vi "ReadBAESdataFromFileVer3.vi"(2 "Factor Size Parameter":dbl=1.0, 3 "Factor Extinction":dbl=1.0 min=0.0 max=150.0 step=1.0, 4 "Factor Ext Uncertainty":dbl=1.0 min=0.0 max=150.0 step=1.0, 5 "file path":path) -> (0 "Extinction data in graph format":T2(array[cluster]), 1 "Extinction ExtinctionUncertainity Size parameter and Number ofS sizes":T3)   [LabVIEW 2013]
uses:
  ReadBaesDataTypeDefinition.ctl
  <vilib>/Platform/storage/lvStorage.llb/_openStorageWithRootAutoDetect.vi
  <vilib>/Platform/storage/lvStorage.llb/xStorage/xStorageSupp/ErrorOut.vi
  <vilib>/Platform/storage/lvStorage.llb/_queryPropPoly.vi
  <vilib>/Platform/storage/lvStorage.llb/_queryPropString.vi
  <vilib>/Platform/storage/lvStorage.llb/_queryGenericObjects.vi
  <vilib>/Platform/storage/lvStorage.llb/_loadAllDouble.vi
  <vilib>/imath/engines/lvmath2/RunTimeEngine/ErrorHandling/NIMS_Finalize Error.vi
  <vilib>/imath/engines/lvmath2/RunTimeEngine/Managers/WorkSpace/UID Generator.vi
  <vilib>/imath/engines/lvmath2/RunTimeEngine/IndexRead/NIMS M(S,$).vi
  <instcachedir>/0/NIMS M(S,$)_F24F360562DE41D8BE234322A2E15C65.lvgen/NIMS M(S,$)_F24F360562DE41D8BE234322A2E15C65_000.vi
  <vilib>/imath/engines/lvmath2/RunTimeEngine/BuiltInFunctions/length/NIMS_length(GV).vi
  <instcachedir>/0/NIMS_length(GV)_08A3D13377FD4E4B96F5795FBF3698FA.lvgen/NIMS_length(GV)_08A3D13377FD4E4B96F5795FBF3698FA_000.vi
  <vilib>/imathl/engines/lvmath/Functions/Error Handling/Create Error.vi
  <vilib>/imath/engines/lvmath2/RunTimeEngine/Managers/SymbolTable/Clear UID.vi
  <vilib>/imath/engines/lvmath2/RunTimeEngine/NodeEndStatement/NIMS_NodeEndStatement_Output.vi
  <instcachedir>/0/NIMS_NodeEndStatement_Output_53EC0D466D134D7ABD903AC30B43404B.lvgen/NIMS_NodeEndStatement_Output_53EC0D466D134D7ABD903AC30B43404B_005.vi
  <instcachedir>/0/NIMS_NodeEndStatement_Output_53EC0D466D134D7ABD903AC30B43404B.lvgen/NIMS_NodeEndStatement_Output_53EC0D466D134D7ABD903AC30B43404B_001.vi
  <instcachedir>/0/NIMS_NodeEndStatement_Output_53EC0D466D134D7ABD903AC30B43404B.lvgen/NIMS_NodeEndStatement_Output_53EC0D466D134D7ABD903AC30B43404B_002.vi
  <vilib>/imath/engines/lvmath2/RunTimeEngine/RangeToken/NIMS_Range.vi
  <instcachedir>/0/NIMS_Range_7481B155BEE341ECA0F59DDB444E2C09.lvgen/NIMS_Range_7481B155BEE341ECA0F59DDB444E2C09_000.vi
  <vilib>/imath/engines/lvmath2/RunTimeSupport/NIMS_Error if Not Equal.vi
  <instcachedir>/0/NIMS_Error if Not Equal_902F5D2649E64F5087A1EF57C55C58AB.lvgen/NIMS_Error if Not Equal_902F5D2649E64F5087A1EF57C55C58AB_001.vi
  <vilib>/imath/engines/lvmath2/RunTimeEngine/IndexRead/NIMS M(S,V).vi
  <instcachedir>/0/NIMS M(S,V)_5C1965D37F59432CA0E9661793EAFE90.lvgen/NIMS M(S,V)_5C1965D37F59432CA0E9661793EAFE90_000.vi
  <vilib>/imath/engines/lvmath2/RunTimeEngine/ErrorHandling/NIMS_Create Error From Enums.vi
  <vilib>/imath/engines/lvmath2/RunTimeEngine/IndexRead/NIMS M(R2,S).vi
  <instcachedir>/0/NIMS M(R2,S)_56813DCFDD5A484292D2195AF15D2BF5.lvgen/NIMS M(R2,S)_56813DCFDD5A484292D2195AF15D2BF5_000.vi
  <vilib>/imath/engines/lvmath2/RunTimeEngine/BuiltInFunctions/repeatmx/NIMS_repeatmx(GM, I32, I32).vi
  <instcachedir>/0/NIMS_repeatmx(GM, I32, I32)_71D32CAC8D434697AB9DA7B55FCB46E4.lvgen/NIMS_repeatmx(GM, I32, I32)_71D32CAC8D434697AB9DA7B55FCB46E4_000.vi
  <vilib>/imath/engines/lvmath2/RunTimeEngine/ArithmeticOperatorToken/NIMS_ArithmeticOperator_rightdiv.vi
  <instcachedir>/0/NIMS_ArithmeticOperator_rightdiv_C75411BD8BC84A93B6F1C8DA359A92EC.lvgen/NIMS_ArithmeticOperator_rightdiv_C75411BD8BC84A93B6F1C8DA359A92EC_004.vi
  <vilib>/imath/engines/lvmath2/RunTimeEngine/RunTimeType/NIMS_RunTimeType_From StrictType (excl LVString).vi
  <instcachedir>/0/NIMS_RunTimeType_From StrictType (excl LVString)_4DEE718D6EB74582AA20236969C084FC.lvgen/NIMS_RunTimeType_From StrictType (excl LVString)_4DEE718D6EB74582AA20236969C084FC_000.vi
  <vilib>/imath/engines/lvmath2/RunTimeEngine/LocalVariableDefStatement/MC_LocalVariableDefStatement_Display.vi
  <vilib>/imath/engines/lvmath2/RunTimeEngine/IndexRead/NIMS M(R2,V).vi
  <instcachedir>/0/NIMS M(R2,V)_2237B96CD57A46B9A0FB7AD48DAEA6E7.lvgen/NIMS M(R2,V)_2237B96CD57A46B9A0FB7AD48DAEA6E7_000.vi
  <vilib>/Platform/storage/Storage.llb/Get Object Info.vi
  <vilib>/Platform/storage/Storage.llb/__closeStorageFromObject.vi
  <vilib>/Platform/storage/lvStorage.llb/xStorage/Open Data Storage/Open Data Storage.xnode
  <vilib>/Platform/storage/lvStorage.llb/xStorage/Read Data/Read Data.xnode
  <vilib>/Platform/storage/lvStorage.llb/xStorage/Close Data Storage/Close Data Storage.xnode
  <vilib>/imath/engines/lvmath2/RunTimeEngine/Managers/SymbolTable/NIMS_WorkSpace.lvlib
panel:
  out "Extinction Data per size":T1(graph)=[{"Ramp Pattern"=[365.01001, 365.56, 366.10001, 366.64999, 367.19, 367.73001, 368.26999, 368.81, 369.35001, 369.89001, 386.09, 386.60001, 387.10999, 387.62, 388.13, 388.63, 389.14001, 389.64999, 390.14999, 390.66, 391.16, 391.67001, 392.17001, 392.67999, 393.17999, 393.67999, 394.17999, 394.67999, 395.19, 395.69, 396.19, 396.69, 397.19, 397.69, 398.19, 398.69, 399.19, 399.67999, 400.17999, 400.67999, 401.17999, 401.67999, 402.17001, 402.67001, 403.17001, 403.66, 404.16, 404.66, 405.14999, 405.64999, 406.14999, 406.64001, 407.14001, 407.64001, 408.13, 408.63, 409.13, 409.62, 410.12, 410.62, 411.10999, 411.60999, 412.10001, 412.60001, 413.10001, 413.60001, 414.09, 414.59, 415.09, 415.59, 416.07999, 416.57999, 417.07999, 417.57999, 418.07999, 418.57999, 419.07999, 419.57999, 420.07999, 420.57999, 421.07999, 421.57999, 422.07999, 422.57999, 423.09, 423.59, 424.09, 424.60001], "Extinction"=[-2.8242922e-13, -9.5446372e-13, -9.5673914e-13, -2.1710713e-12, -3.0653965e-12, -3.5744682e-12, -2.7968654e-12, -2.494626e-12, -1.8658978e-12, -2.7078036e-12, 1.199962e-09, 1.2044283e-09, 1.1869159e-09, 1.1971283e-09, 1.1743045e-09, 1.1673239e-09, 1.1844579e-09, 1.1774074e-09, 1.1781032e-09, 1.1685674e-09, 1.1821694e-09, 1.1679153e-09, 1.1804325e-09, 1.1549264e-09, 1.1582446e-09, 1.1719666e-09, 1.1561709e-09, 1.1576946e-09, 1.1596397e-09, 1.1522512e-09, 1.1499967e-09, 1.1519218e-09, 1.1412127e-09, 1.136586e-09, 1.1347415e-09, 1.1384925e-09, 1.1290678e-09, 1.134521e-09, 1.125919e-09, 1.1187079e-09, 1.1216958e-09, 1.1213084e-09, 1.1191187e-09, 1.1248569e-09, 1.1156328e-09, 1.1128937e-09, 1.1153232e-09, 1.1142656e-09, 1.1032915e-09, 1.1037591e-09, 1.0994153e-09, 1.0982592e-09, 1.0898938e-09, 1.0945469e-09, 1.090964e-09, 1.0935359e-09, 1.0873367e-09, 1.0829221e-09, 1.0798286e-09, 1.0773584e-09, 1.0711578e-09, 1.0749976e-09, 1.0730125e-09, 1.0733134e-09, 1.0667034e-09, 1.0626963e-09, 1.0597497e-09, 1.0538669e-09, 1.056263e-09, 1.0531479e-09, 1.0517495e-09, 1.0454831e-09, 1.0547482e-09, 1.0485262e-09, 1.0436499e-09, 1.042629e-09, 1.0315969e-09, 1.0291459e-09, 1.0254163e-09, 1.0385639e-09, 1.0386701e-09, 1.0280848e-09, 1.0382387e-09, 1.0251714e-09, 1.0107518e-09, 1.0066801e-09, 1.0073331e-09, 1.0244581e-09]}, {"Ramp Pattern"=[365.01001, 365.01001, 365.01001, 365.56, 365.56, 365.56, 366.10001, 366.10001, 366.10001, 366.64999, 366.64999, 366.64999, 367.19, 367.19, 367.19, 367.73001, 367.73001, 367.73001, 368.26999, 368.26999, 368.26999, 368.81, 368.81, 368.81, 369.35001, 369.35001, 369.35001, 369.89001, 369.89001, 369.89001, 386.09, 386.09, 386.09, 386.60001, 386.60001, 386.60001, 387.10999, 387.10999, 387.10999, 387.62, 387.62, 387.62, 388.13, 388.13, 388.13, 388.63, 388.63, 388.63, 389.14001, 389.14001, 389.14001, 389.64999, 389.64999, 389.64999, 390.14999, 390.14999, 390.14999, 390.66, 390.66, 390.66, 391.16, 391.16, 391.16, 391.67001, 391.67001, 391.67001, 392.17001, 392.17001, 392.17001, 392.67999, 392.67999, 392.67999, 393.17999, 393.17999, 393.17999, 393.67999, 393.67999, 393.67999, 394.17999, 394.17999, 394.17999, 394.67999, 394.67999, 394.67999, 395.19, 395.19, 395.19, 395.69, 395.69, 395.69, 396.19, 396.19, 396.19, 396.69, 396.69, 396.69, 397.19, 397.19, 397.19, 397.69, 397.69, 397.69, 398.19, 398.19, 398.19, 398.69, 398.69, 398.69, 399.19, 399.19, 399.19, 399.67999, 399.67999, 399.67999, 400.17999, 400.17999, 400.17999, 400.67999, 400.67999, 400.67999, 401.17999, 401.17999, 401.17999, 401.67999, 401.67999, 401.67999, 402.17001, 402.17001, 402.17001, 402.67001, 402.67001, 402.67001, 403.17001, 403.17001, 403.17001, 403.66, 403.66, 403.66, 404.16, 404.16, 404.16, 404.66, 404.66, 404.66, 405.14999, 405.14999, 405.14999, 405.64999, 405.64999, 405.64999, 406.14999, 406.14999, 406.14999, 406.64001, 406.64001, 406.64001, 407.14001, 407.14001, 407.14001, 407.64001, 407.64001, 407.64001, 408.13, 408.13, 408.13, 408.63, 408.63, 408.63, 409.13, 409.13, 409.13, 409.62, 409.62, 409.62, 410.12, 410.12, 410.12, 410.62, 410.62, 410.62, 411.10999, 411.10999, 411.10999, 411.60999, 411.60999, 411.60999, 412.10001, 412.10001, 412.10001, 412.60001, 412.60001, 412.60001, 413.10001, 413.10001, 413.10001, 413.60001, 413.60001, 413.60001, 414.09, 414.09, 414.09, 414.59, 414.59, 414.59, 415.09, 415.09, 415.09, 415.59, 415.59, 415.59, 416.07999, 416.07999, 416.07999, 416.57999, 416.57999, 416.57999, 417.07999, 417.07999, 417.07999, 417.57999, 417.57999, 417.57999, 418.07999, 418.07999, 418.07999, 418.57999, 418.57999, 418.57999, 419.07999, 419.07999, 419.07999, 419.57999, 419.57999, 419.57999, 420.07999, 420.07999, 420.07999, 420.57999, 420.57999, 420.57999, 421.07999, 421.07999, 421.07999, 421.57999, 421.57999, 421.57999, 422.07999, 422.07999, 422.07999, 422.57999, 422.57999, 422.57999, 423.09, 423.09, 423.09, 423.59, 423.59, 423.59, 424.09, 424.09, 424.09, 424.60001, 424.60001, 424.60001], "Extinction"=[nan, 5.63555038e-12, -6.20040882e-12, nan, 4.42688488e-12, -6.33581232e-12, nan, 4.44172376e-12, -6.35520204e-12, nan, 3.1925879e-12, -7.5347305e-12, nan, 1.9136571e-12, -8.044450099999999e-12, nan, 1.7542992000000003e-12, -8.9032356e-12, nan, 2.3729171999999995e-12, -7.966648e-12, nan, 2.7093124e-12, -7.6985644e-12, nan, 4.4583185e-12, -8.1901141e-12, nan, 2.9758349000000003e-12, -8.3914421e-12, nan, 1.3537115500000002e-09, 1.04621245e-09, nan, 1.33050989e-09, 1.0783467100000001e-09, nan, 1.29980645e-09, 1.07402535e-09, nan, 1.30703543e-09, 1.0872211700000001e-09, nan, 1.263323188e-09, 1.085285812e-09, nan, 1.257682822e-09, 1.0769649780000001e-09, nan, 1.257997803e-09, 1.110917997e-09, nan, 1.258281811e-09, 1.0965329889999999e-09, nan, 1.249724367e-09, 1.106482033e-09, nan, 1.233311541e-09, 1.1038232590000001e-09, nan, 1.242856071e-09, 1.1214827290000002e-09, nan, 1.220968997e-09, 1.114861603e-09, nan, 1.237850674e-09, 1.123014326e-09, nan, 1.20776521e-09, 1.1020875899999999e-09, nan, 1.207318623e-09, 1.1091705769999999e-09, nan, 1.219534456e-09, 1.124398744e-09, nan, 1.206780784e-09, 1.105561016e-09, nan, 1.2016583529999999e-09, 1.113730847e-09, nan, 1.202722643e-09, 1.1165567570000001e-09, nan, 1.193639166e-09, 1.110863234e-09, nan, 1.190472677e-09, 1.1095207229999998e-09, nan, 1.192674486e-09, 1.1111691140000001e-09, nan, 1.1818626490000002e-09, 1.100562751e-09, nan, 1.1711783190000001e-09, 1.101993681e-09, nan, 1.171442972e-09, 1.0980400280000001e-09, nan, 1.1742146020000001e-09, 1.102770398e-09, nan, 1.1647996130000001e-09, 1.093335987e-09, nan, 1.1680687030000001e-09, 1.100973297e-09, nan, 1.158754071e-09, 1.0930839290000001e-09, nan, 1.150347064e-09, 1.0870687359999998e-09, nan, 1.153138513e-09, 1.0902530870000001e-09, nan, 1.1536706730000001e-09, 1.088946127e-09, nan, 1.152280031e-09, 1.085957369e-09, nan, 1.155661193e-09, 1.094052607e-09, nan, 1.147199119e-09, 1.0840664810000001e-09, nan, 1.145071783e-09, 1.080715617e-09, nan, 1.147246497e-09, 1.083399903e-09, nan, 1.143375044e-09, 1.0851561559999999e-09, nan, 1.1348594220000001e-09, 1.071723578e-09, nan, 1.135517436e-09, 1.072000764e-09, nan, 1.125704434e-09, 1.0731261660000001e-09, nan, 1.127667266e-09, 1.0688511340000001e-09, nan, 1.117893049e-09, 1.061894551e-09, nan, 1.126185515e-09, 1.062908285e-09, nan, 1.1200817459999999e-09, 1.061846254e-09, nan, 1.1247833070000001e-09, 1.062288493e-09, nan, 1.117086625e-09, 1.057586775e-09, nan, 1.11416822e-09, 1.0516759800000001e-09, nan, 1.111104457e-09, 1.048552743e-09, nan, 1.107725349e-09, 1.046991451e-09, nan, 1.104137273e-09, 1.038178327e-09, nan, 1.107764944e-09, 1.042230256e-09, nan, 1.106480232e-09, 1.039544768e-09, nan, 1.110412925e-09, 1.0362138749999999e-09, nan, 1.1036413210000002e-09, 1.029765479e-09, nan, 1.099794992e-09, 1.0255976079999999e-09, nan, 1.098809091e-09, 1.0206903090000001e-09, nan, 1.094440483e-09, 1.013293317e-09, nan, 1.09649886e-09, 1.01602714e-09, nan, 1.095379445e-09, 1.010916355e-09, nan, 1.095129175e-09, 1.008369825e-09, nan, 1.0888327469999999e-09, 1.002133453e-09, nan, 1.105700682e-09, 1.0037957179999999e-09, nan, 1.096226079e-09, 1.0008263209999998e-09, nan, 1.090656791e-09, 9.96643009e-10, nan, 1.096478637e-09, 9.88779363e-10, nan, 1.08555377e-09, 9.7764003e-10, nan, 1.0987320770000001e-09, 9.59559723e-10, nan, 1.099013116e-09, 9.51819484e-10, nan, 1.115469798e-09, 9.61658002e-10, nan, 1.121745799e-09, 9.55594401e-10, nan, 1.1148866849999999e-09, 9.41282915e-10, nan, 1.14595311e-09, 9.305242899999999e-10, nan, 1.13382451e-09, 9.165182899999999e-10, nan, 1.15459483e-09, 8.6690877e-10, nan, 1.14573256e-09, 8.676276399999999e-10, nan, 1.19507904e-09, 8.1958716e-10, nan, 1.2450424e-09, 8.038738e-10]}, ...(18 in all)]
  out "WaveLengths 2":dbl[](array[numeric])
  out "Sizes":dbl[](array[numeric])
  in  "Extinction ExtinctionUncertainity Size parameter and Number ofS sizes 2":T3
  out "Signal":dbl[][](array[numeric])
  out "GeometricCrossSection":dbl[](array[numeric])
  out "Number Of Sizes":dbl
  out "SizeParameter":dbl[][](array[numeric])
  in  "Slide":i16(slide) scale=0.0..100.0
  out "Extinction Graph":cluster{"Extinction":dbl[], "Sizes":dbl[]}[](graph)
  out "ExtinctionUncertainty":dbl[][](array[numeric])
  out "Extinction":dbl[][](array[numeric])
  out "WaveLengths":dbl[](array[numeric])
  out "error out":errorcluster
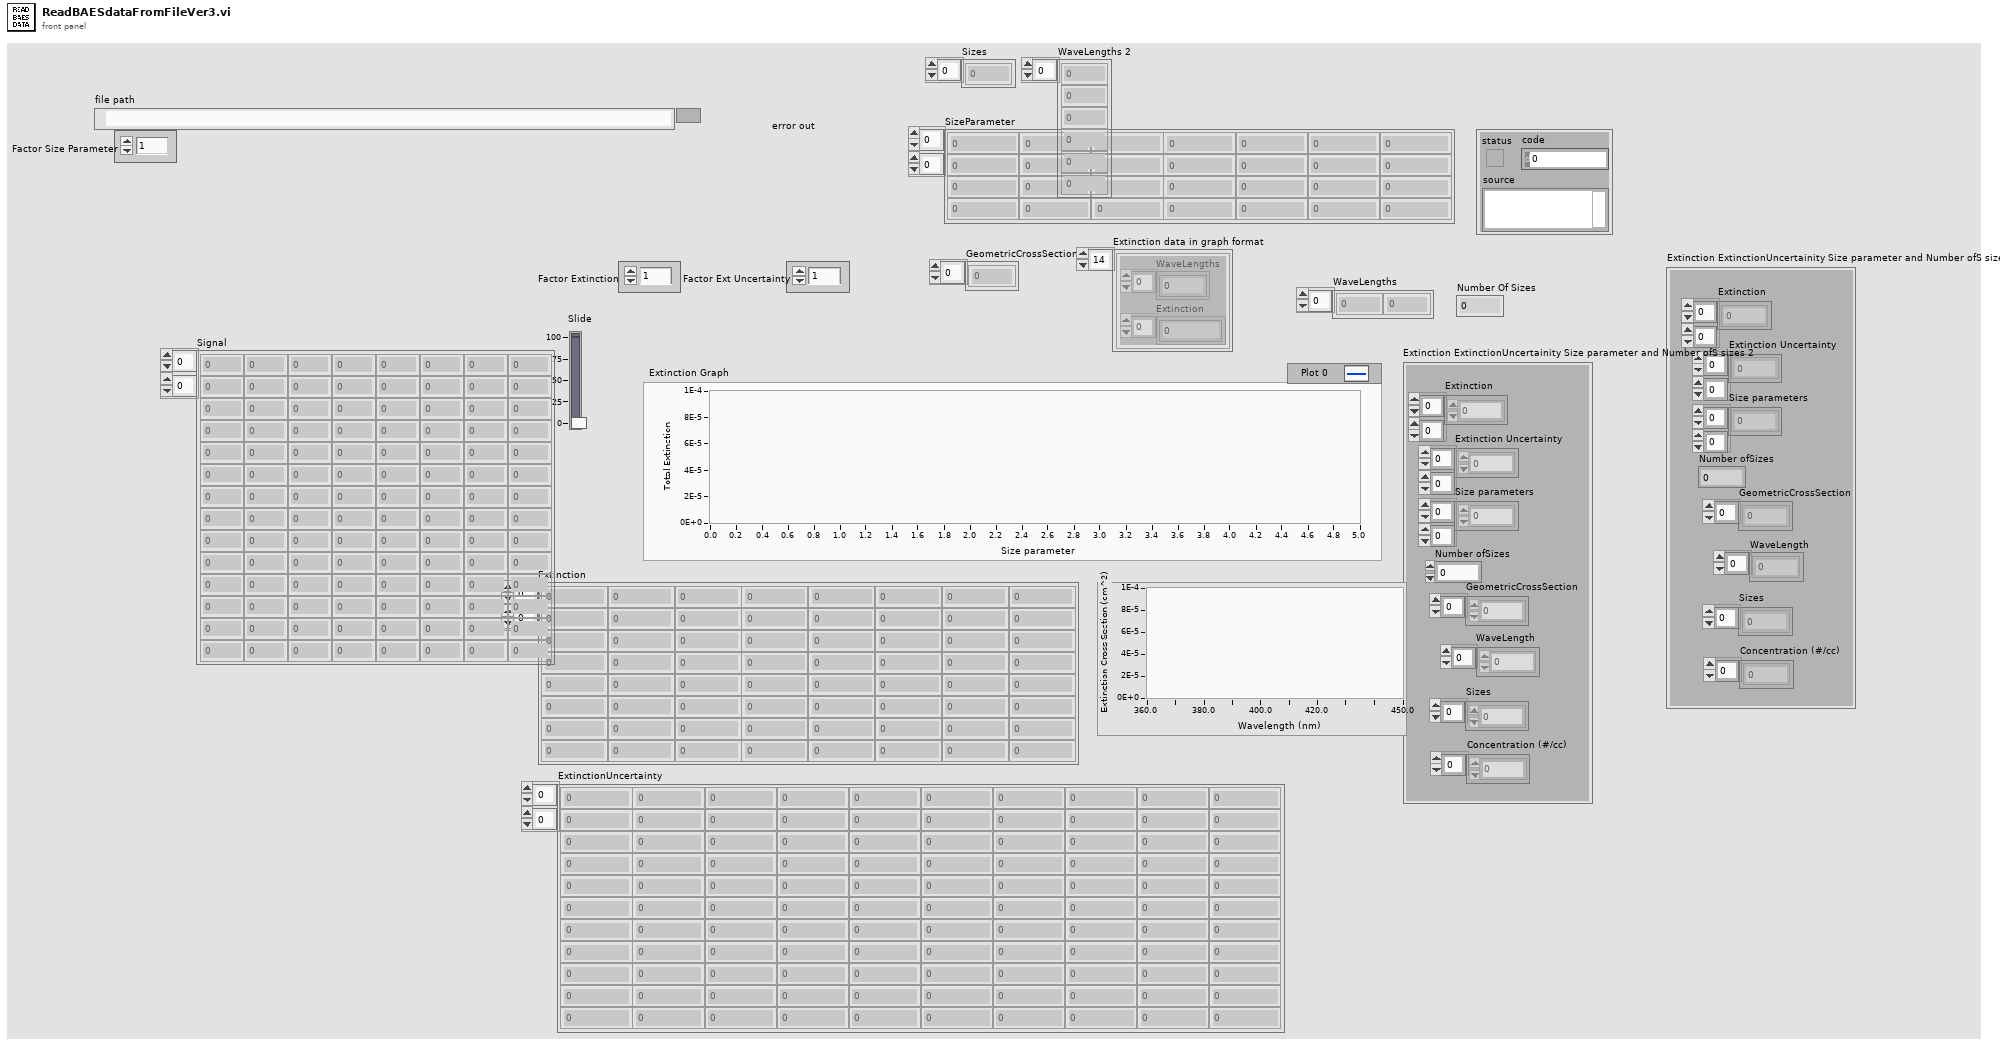
[diagram p1: front panel]
types:
  T1 = cluster{"Ramp Pattern":dbl[], "Extinction":dbl[]}[]
  T2 = cluster{"WaveLengths":dbl[], "Extinction":dbl[]}[]
  T3 = typedef "ReadBaesDataTypeDefinition.ctl" = cluster{"Extinction":dbl[][], "Extinction Uncertainty":dbl[][], "Size parameters":dbl[][], "Number ofSizes":dbl, "GeometricCrossSection":dbl[], "WaveLength":dbl[], "Sizes":dbl[], "Concentration (#/cc)":dbl[]}
  T4 = enum16{"open", "open or create", "create or replace", "create", "open (read only)"}
  T5 = cluster{"SizeParameter":dbl[], "Extinction":dbl[]}
  T6 = cluster{"SizeParameter":dbl[], "Extinction":dbl[]}[]
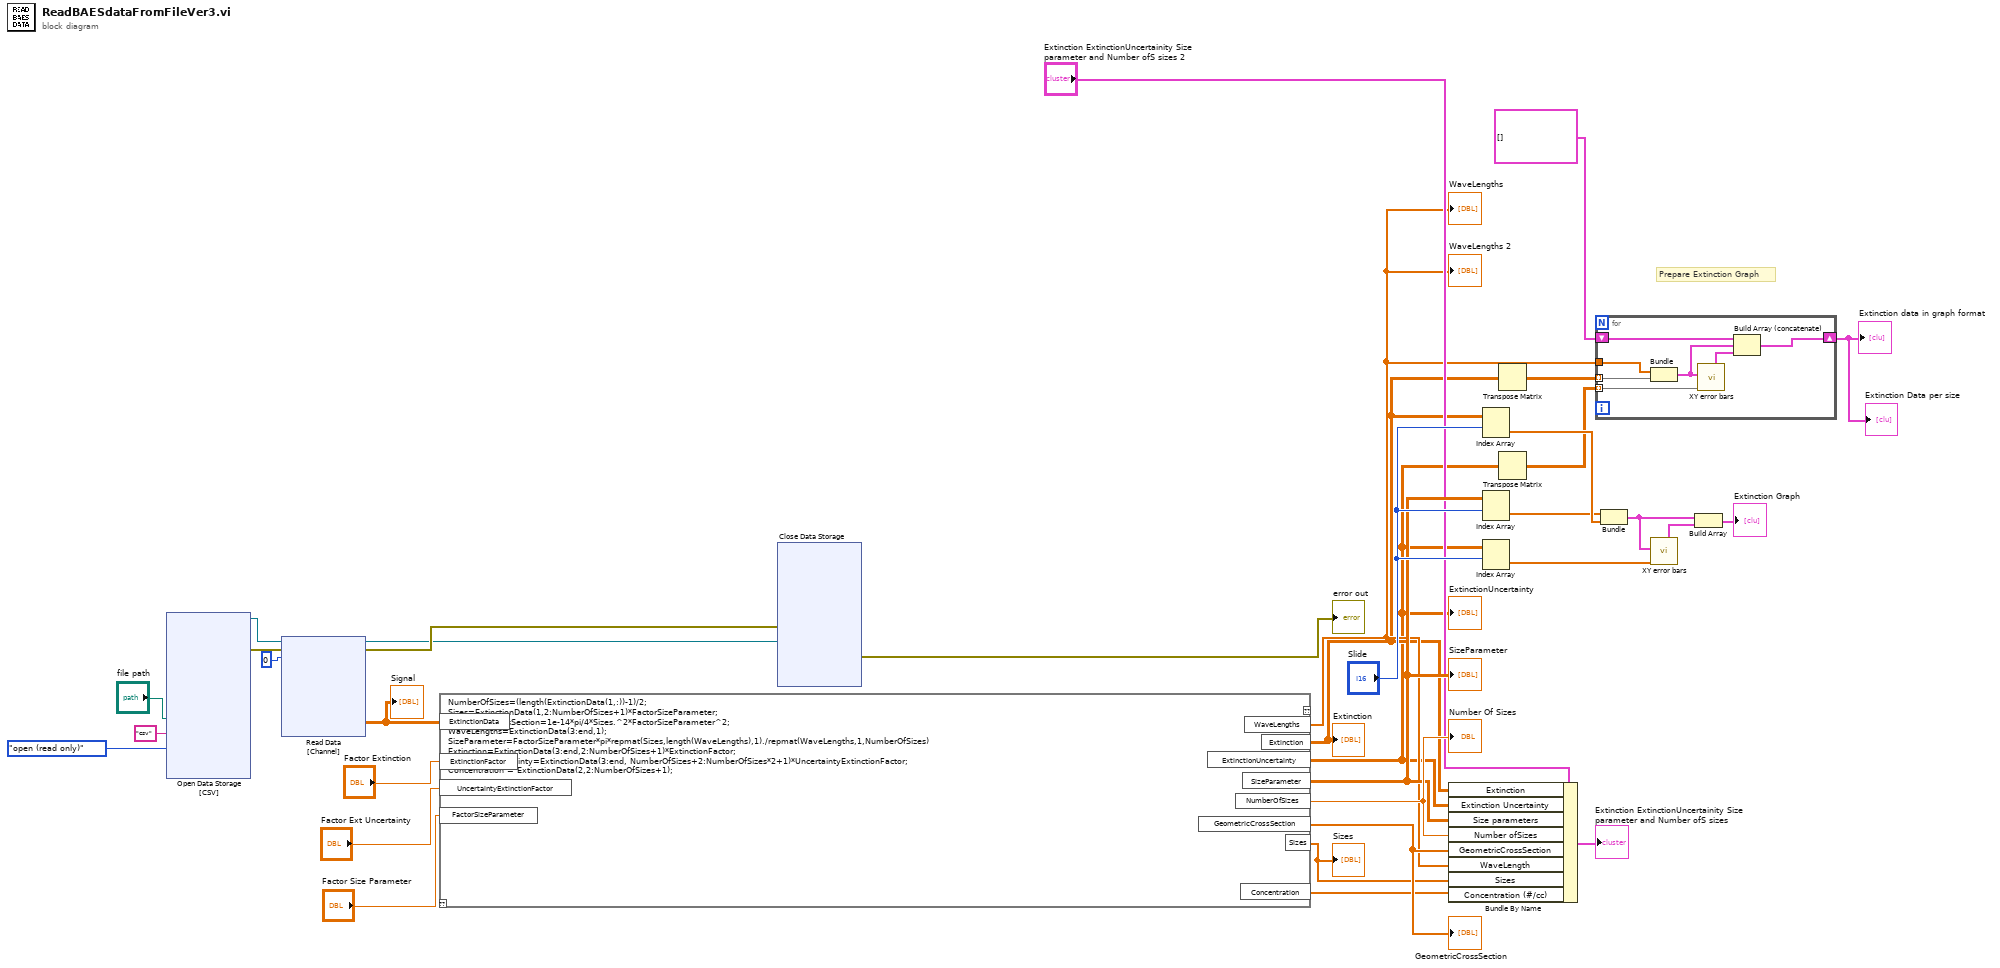
[diagram p0: block diagram]
diagram:
  # "Prepare Extinction Graph"
  n1 = xnode "Open Data Storage\n[CSV]"("file path"="file path", "DataPlugin name"="csv", "function (open:0)"=T4."open (read only)") -> ("storage refnum (file)"=w34:refnum<k20>, "error out"=w33:errorcluster)  [unwired: 2 in, 1 out]
  n2 = xnode "Read Data\n[Channel]"("storage refnum (file)"=w34, "error in"=w33, "index"=0) -> ("Signal"=w20:dbl[][], "storage refnum (file) out"=w28:refnum<k20>, "error out"=w32:errorcluster)  [unwired: 1 in, 1 out]
  "Signal" <- w20
  n3 = mathscript code="NumberOfSizes=(length(ExtinctionData(1,:))-1)/2;\nSizes=ExtinctionData(1,2:NumberOfSizes+1)*FactorSizeParameter;\nGeometricCrossSection=1e-14*pi/4*Sizes.^2*FactorSizeParameter^2;\nWaveLengths=ExtinctionData(3:end,1);\nSizeParameter=FactorSizeParameter*pi*repmat(Sizes,length(WaveLengths),1)./repmat(WaveLengths,1,NumberOfSizes)\nExtinction=ExtinctionData(3:end,2:NumberOfSizes+1)*ExtinctionFactor;\nExtinctionUncertainty=ExtinctionData(3:end, NumberOfSizes+2:NumberOfSizes*2+1)*UncertaintyExtinctionFactor;\nConcentration = ExtinctionData(2,2:NumberOfSizes+1);"("ExtinctionData"=w20, "ExtinctionFactor"="Factor Extinction", "UncertaintyExtinctionFactor"="Factor Ext Uncertainty", "FactorSizeParameter"="Factor Size Parameter") -> ("WaveLengths"=w8:dbl[], "Extinction"=w6:dbl[][], "ExtinctionUncertainty"=w4:dbl[][], "SizeParameter"=w15:dbl[][], "NumberOfSizes"=w17:dbl, "GeometricCrossSection"=w16:dbl[], "Sizes"=w12:dbl[], "Concentration"=w2:dbl[])  [unwired: 1 in, 1 out]
  "WaveLengths" <- w8
  "Extinction" <- w6
  "ExtinctionUncertainty" <- w4
  "SizeParameter" <- w15
  "Number Of Sizes" <- w17
  "GeometricCrossSection" <- w16
  "Sizes" <- w12
  "WaveLengths 2" <- w8
  n4 = xnode "Close Data Storage\n"("error in (no error)"=w32, "storage refnum (file)"=w28) -> ("error out"=→"error out":errorcluster)  [unwired: 1 out]
  n5 = Bundle By Name(cluster="Extinction ExtinctionUncertainity Size parameter and Number ofS sizes 2", "Extinction"=w6, "Extinction Uncertainty"=w4, "Size parameters"=w15, "Number ofSizes"=w17, "GeometricCrossSection"=w16, "WaveLength"=w8, "Sizes"=w12, "Concentration (#/cc)"=w2) -> (→"Extinction ExtinctionUncertainity Size parameter and Number ofS sizes":T3)
  n6 = Index Array(array=w6, index (row)="Slide") -> (element=w23:dbl[])  [unwired: 1 in]
  n7 = Index Array(array=w15, index (row)="Slide") -> (element=w21:dbl[])  [unwired: 1 in]
  n8 = Index Array(array=w4, index (row)="Slide") -> (element=w27:dbl[])  [unwired: 1 in]
  n9 = Transpose Matrix(1:w6) -> (0:w5:dbl[][])
  n10 = Transpose Matrix(1:w4) -> (0:w3:dbl[][])
  n11 = for {
    tunnel: w5 -> [w41] mode=indexing
    tunnel: w3 -> [w39] mode=indexing
    tunnel: w8 -> [w40]
    shift-right: [w36] -> w1
    shift-left: T2 [] ("appended array") -> [w35]
    n12 = Bundle("WaveLengths"=w40, "Extinction"=w41) -> (w37:cluster{"WaveLengths":dbl[], "Extinction":dbl[]})  [unwired: 1 in]
    n13 = call "XY error bars.vi"("XY plot"=w37, "Yerror"=w39) -> ("Y error bars"=w38:cluster{dbl[], dbl[]})  [unwired: 6 in, 2 out]
    n14 = Build Array (concatenate)(w35, w37, w38) -> (w36:T2)
  }
  "Extinction data in graph format" <- w1
  "Extinction Data per size" <- w1
  n15 = Bundle("SizeParameter"=w21, "Extinction"=w23) -> (w26:T5)  [unwired: 1 in]
  n16 = call "XY error bars.vi"("XY plot"=w26, "Yerror"=w27) -> ("Y error bars"=w25:cluster{dbl[], dbl[]})  [unwired: 6 in, 2 out]
  n17 = Build Array(w26, w25) -> (→"Extinction Graph":T6)
